vi "Self-Test.vi"(0 "VISA Resource Name":refnum<visa-resource-name>, 11 "error in (no error)":errorcluster) -> (4 "VISA Resource Name Out":refnum<visa-resource-name>, 8 "Self-Test Error":u32, 10 "Self-Test Response":string, 15 "error out":errorcluster)   [LabVIEW 2016, in "Agilent 34970.lvlib"]
doc: "This VI causes the instrument to perform a self-test and returns the results. A numeric indicator indicates if the instrument passed all self-tests, and a string indicator contains the instrument's reponse."
uses:
  Agilent 34970.lvlib
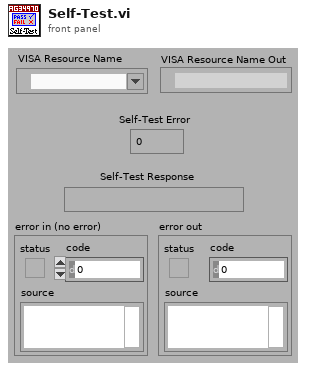
[diagram p1: front panel]
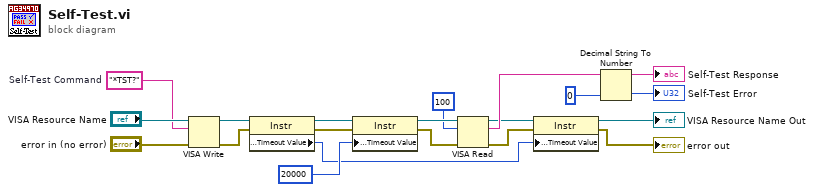
[diagram p0: block diagram]
diagram:
  w3 = "*TST?"  # Self-Test Command
  n1 = VISA Write(VISA resource name="VISA Resource Name", write buffer=w3, error in (no error)="error in (no error)") -> (VISA resource name out=w12:refnum<visa-resource-name>, error out=w13:errorcluster)  [unwired: 1 out]
  n2 = property class="Instr"(reference=w12, error in=w13) -> (reference out=w11:refnum<visa-resource-name>, error out=w10:errorcluster, "General Settings:Timeout Value"=w6:u32)
  n3 = property class="Instr"(reference=w11, error in=w10, "General Settings:Timeout Value"=u32 20000 ("Tmo Value")) -> (reference out=w16:refnum<visa-resource-name>, error out=w15:errorcluster)
  n4 = VISA Read(VISA resource name=w16, byte count=u32 100 ("byte count (0)"), error in (no error)=w15) -> (VISA resource name out=w7:refnum<visa-resource-name>, read buffer=w9:string, error out=w8:errorcluster)  [unwired: 1 out]
  "Self-Test Response" <- w9
  n5 = property class="Instr"(reference=w7, error in=w8, "General Settings:Timeout Value"=w6) -> (reference out=→"VISA Resource Name Out":refnum<visa-resource-name>, error out=→"error out":errorcluster)
  n6 = Decimal String To Number(string=w9, default (0L)=u32 0 ("Default (0L)")) -> (number=→"Self-Test Error":u32)  [unwired: 1 in, 1 out]
